vi "read tree ref.vi"(8 "error in (no error)":errorcluster, 11 "alias-tree in":refnum<class "alias-tree.lvclass">) -> (0 "error out":errorcluster, 1 "tree ref":refnum<k24>, 3 "alias-tree out":refnum<class "alias-tree.lvclass">)   [LabVIEW 2017, in "vs-tree-utility.lvlib" / "alias-tree.lvclass"]
uses:
  alias-tree.lvclass
  NationalInstruments.VeriStand.SystemStorageUI
  alias-tree.lvclass/alias-tree.ctl
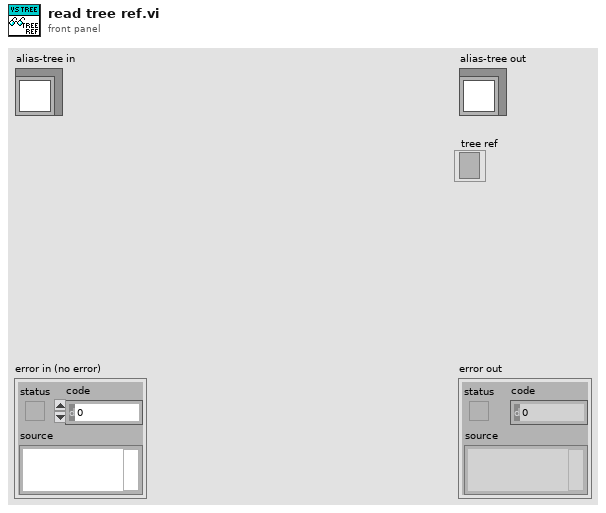
[diagram p1: front panel]
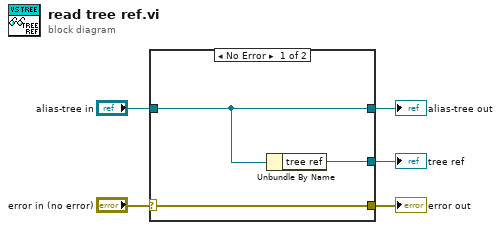
[diagram p0: block diagram]
diagram:
  n1 = case shown="No Error" "error in (no error)" {
    selector: "error in (no error)" -> [w8 w10]
    tunnel: [w8 w10] -> w4
    tunnel: [w7 w9] -> w2
    tunnel: "alias-tree in" -> [w7 w9]
    tunnel: [w6 _] -> w1
    frame No Error {
      n2 = Unbundle By Name(w7) -> ("tree ref"=w6:refnum<k24>)
    }
    frame Error {
    }
  }
  "error out" <- w4
  "alias-tree out" <- w2
  "tree ref" <- w1
